vi "macro_LinearSystemLoop_DiffDrv_Model_Execute.vi"() -> ()   [LabVIEW 2019, in "Trajectory_Library.lvlib"]
uses:
  Trajectory_Library.lvlib
  Enum/DCMOTOR_TYPES_ENUM.ctl
  LinearSystemId_CreateDriveTrainVelocitySystem.vi
  DCMotor_PickMotor_OLD.vi
  LinearSystem_New.vi
  MatBuilder_Create.vi
  MatBuilder_Fill.vi
  MatrixHelper_Zero.vi
  DCMotor_GetCIM.vi
  DCMotor_GetAndymark9015.vi
  DCMotor_GetAndymarkRs775_125.vi
  DCMotor_GetBag.vi
  DCMotor_GetBanebotsRs550.vi
  DCMotor_GetBanebotsRs775.vi
  DCMotor_GetFalcon500.vi
  DCMotor_GetMiniCIM.vi
  DCMotor_GetNEO.vi
  DCMotor_GetNEO550.vi
  DCMotor_GetRomiBuiltIn.vi
  DCMotor_GetVex775Pro.vi
  VI/DCMotor_GetAndymarkAM2235A.vi
  VI/DCMotor_GetAndymarkAM3493.vi
  MatrixHelper_CoerceSize.vi
  DCMotor_New.vi
  VI/Units_RotationsPerMinuteToRadiansPerSecond.vi
panel:
  out "Left Motor Dmd":dbl
  out "Right Motor Dmd":dbl
  in  "Left Vel SP m/s":dbl
  in  "Right Vel SP m/s":dbl
  in  "Left Vel PV m/s":dbl
  in  "Right Vel PV m/s":dbl
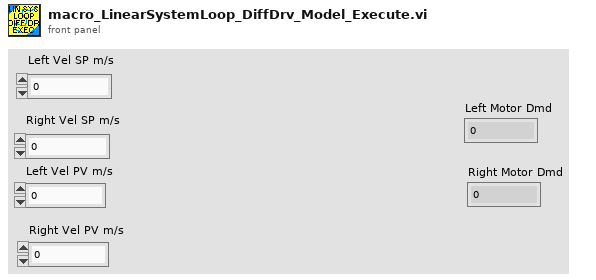
[diagram p1: front panel]
types:
  T1 = typedef "Trajectory_Library.lvlib/DCMOTOR_TYPES_ENUM.ctl" = enum16{"CIM", "AndyMark 9015", "Andy Mark RS 775 125", "Bag", "BaneBots RS 550", "BaneBots RS 775", "Falcon 500", "Mini CIM", "NEO", "NEO 550", "Romi BuiltIn", "Vex 775 Pro", "Snow Blower AM 2235A", "Bosch Seat AM 3493"}
  T2 = typedef "Trajectory_Library.lvlib/LINEAR_SYSTEM.ctl" = cluster{"m_A":T3, "m_B":T3, "m_C":T3, "m_D":T3, "States":i32, "Inputs":i32, "Outputs":i32}
  T3 = typedef "NI_Matrix.lvlib/RealMatrix.ctl" = dbl[][]
  T4 = typedef "Trajectory_Library.lvlib/LINEAR_SYSTEM_LOOP_DIFF_DRV_CTRL_PARAMS.CTL" = cluster{"Left Vel Model Std Dev m/s":dbl, "Left Vel Meas Std Dev m/s":dbl, "Left Vel Ctrl Tol m/s":dbl, "Max Control Effort":dbl, "Right Vel Ctrl Tol m/s":dbl, "Right Vel Meas Std Dev m/s":dbl, "Right Vel Model Std Dev m/s":dbl}
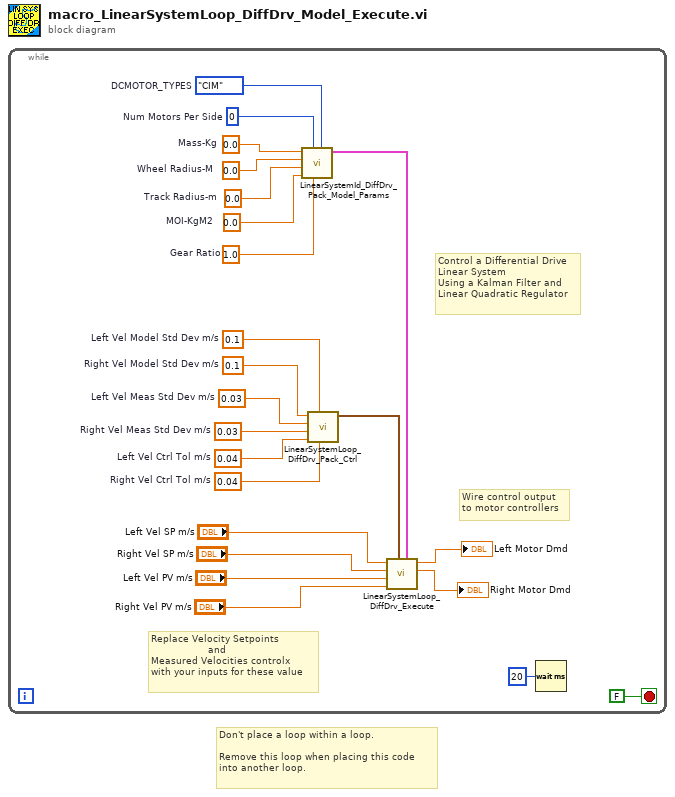
[diagram p0: block diagram]
diagram:
  # "Don't place a loop within a loop.\n \nRemove this loop when placing this code\ninto another loop."
  n1 = while {
    stop <- FALSE stop-if-true
    w7 = 0.1  # Right Vel Model Std Dev m/s
    w8 = 0.03  # Left Vel Meas Std Dev m/s
    w9 = 0.03  # Right Vel Meas Std Dev m/s
    w10 = 0.04  # Left Vel Ctrl Tol m/s
    w11 = 0.1  # Left Vel Model Std Dev m/s
    w12 = 0.04  # Right Vel Ctrl Tol m/s
    w13 = 0.0  # Mass-Kg
    w14 = 0.0  # Wheel Radius-M
    w15 = 0.0  # Track Radius-m
    w16 = 0.0  # MOI-KgM2
    w17 = 0  # Num Motors Per Side
    w18 = 1.0  # Gear Ratio
    w19 = DCMOTOR_TYPES_ENUM."CIM"  # DCMOTOR_TYPES
    # "Wire control output\nto motor controllers"
    # "Replace Velocity Setpoints \n                   and \nMeasured Velocities controlx\nwith your inputs for these value"
    # "Control a Differential Drive\nLinear System\nUsing a Kalman Filter and \nLinear Quadratic Regulator"
    n2 = call "LinearSystemId_DiffDrv_Pack_Model_Params.vi"("DCMOTOR_TYPES"=w19, "Gear Ratio"=w18, "Num Motors Per Side"=w17, "MOI-KgM2"=w16, "Track Radius-m"=w15, "Wheel Radius-M"=w14, "Mass-Kg"=w13) -> ("DiffDrv_LinearSystem"=w20:T2)  [unwired: 4 in]
    n3 = call "LinearSystemLoop_DiffDrv_Pack_Ctrl.vi"("Right Vel Ctrl Tol m/s"=w12, "Left Vel Model Std Dev m/s"=w11, "Left Vel Ctrl Tol m/s"=w10, "Right Vel Meas Std Dev m/s"=w9, "Left Vel Meas Std Dev m/s"=w8, "Right Vel Model Std Dev m/s"=w7) -> ("LinearSystemLoop_DiffDrv_Ctrl_Params"=w21:T4)  [unwired: 5 in]
    n4 = call "LinearSystemLoop_DiffDrv_Execute.vi"("Linear System"=w20, "LinearSystemLoop_DiffDrv_Control_Params"=w21, "Right Vel PV m/s"="Right Vel PV m/s", "Left Vel PV m/s"="Left Vel PV m/s", "Right Vel SP m/s"="Right Vel SP m/s", "Left Vel SP m/s"="Left Vel SP m/s") -> ("Right Motor Dmd"=→"Right Motor Dmd":dbl, "Left Motor Dmd"=→"Left Motor Dmd":dbl)  [unwired: 1 in, 3 out]
    n5 = Wait (ms)(milliseconds to wait=u32 20) -> ()  [unwired: 1 out]
  }
